vi "C2F converter.vi"() -> ()   [LabVIEW 2018]
panel:
  out "High Temp":bool
  in  "?":bool
  out "In Farenheit":dbl(slide) scale=0.0..100.0
  in  "In Celsius":dbl(knob) scale=0.0..100.0
  # "C2F Converter"
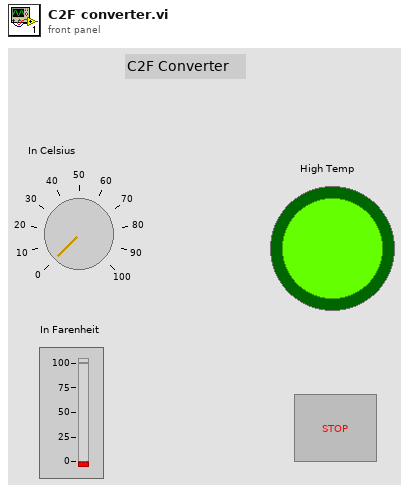
[diagram p1: front panel]
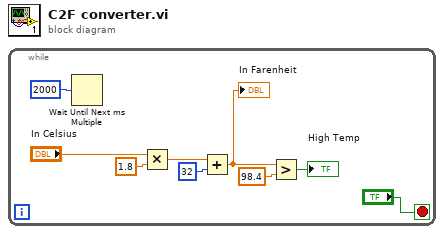
[diagram p0: block diagram]
diagram:
  n1 = while {
    stop <- "?" stop-if-true
    n2 = Wait Until Next ms Multiple(millisecond multiple=u32 2000) -> ()  [unwired: 1 out]
    n3 = Multiply(x="In Celsius", y=1.8) -> (x*y=w6:dbl)
    n4 = Add(x=w6, y=32) -> (x+y=w5:dbl)
    "In Farenheit" <- w5
    n5 = Greater?(x=w5, y=98.4) -> (0:→"High Temp":bool)
  }
